vi "Apply Theme To Buttons.vi"(7 "Override Root With (Empty)":string, 8 "Error In":errorcluster, 9 "Window Element":T1, 10 "Buttons Ref":refnum<vi>[](array[refnum]), 11 "ini Theme in":refnum<class "ini Theme.lvclass">) -> (0 "Error Out":errorcluster, 3 "ini Theme out":refnum<class "ini Theme.lvclass">)   [LabVIEW 2021, in "Appearance Actor.lvlib" / "ini Theme.lvclass"]
doc: "Apply theme to <B>Buttons</B> (Bool Reference Array). <B>Window Element</B> enum tells where it is on the window. <B>Override Root With</B> allows to override styling used for main window components."
uses:
  ini Theme.lvclass
  Generic Theme/API/Typedefs/Window Element--enum.ctl
  Generic Theme/API/Typedefs/Theme Control Property--enum.ctl
  ini Theme.lvclass/ini Theme.ctl
  f5176d82-9832-41ee-acb3-f85e09ee67a5.vi
  f5176d82-9832-41ee-acb3-f85e09ee67a5.vi/e124eda1-1651-4d76-919f-d33a8200b27b.vi
  f5176d82-9832-41ee-acb3-f85e09ee67a5.vi/2055fcb7-c480-499a-9c31-028cc01b484e.vi
  Generic Theme/API/Utilities/Theme Entry Enum To String.vi
  Generic Theme/API/Utilities/U32 Color To Hexa String.vi
  <vilib>/Utility/config.llb/Read Key.vi
  <vilib>/Utility/config.llb/Read Key (String).vi
  <vilib>/Utility/config.llb/NI_LVConfig.lvlib
  Generic Theme/Generic Theme.lvclass
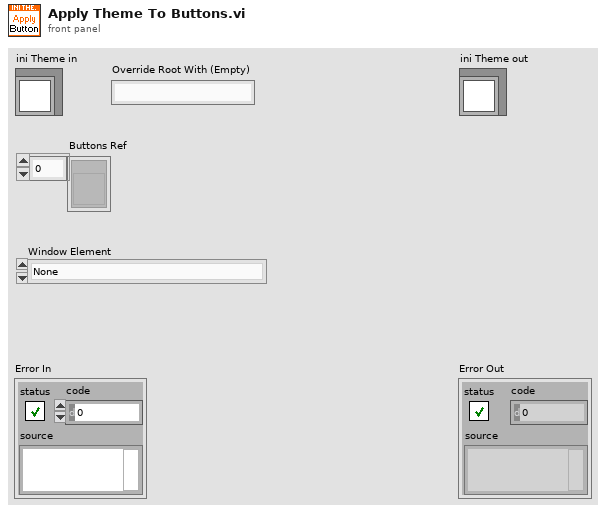
[diagram p1: front panel]
types:
  T1 = typedef "Appearance Actor.lvlib/Generic Theme.lvclass/Window Element--enum.ctl" = enum16{"None", "TB", "SM", "BP", "SB"}
  T2 = typedef "Appearance Actor.lvlib/Generic Theme.lvclass/Theme Control Property--enum.ctl" = enum16{"None", "Button.FalseFillColor", "Button.FalseOutlineColor", "Button.FalseToTrueFillColor", "Button.FalseToTrueOutlineColor", "Button.HoverFalseFillColor", "Button.HoverFalseOutlineColor", "Button.HoverTrueFillColor", "Button.HoverTrueOutlineColor", "Button.TrueFillColor", "Button.TrueOutlineColor", "Button.TrueToFalseFillColor", "Button.TrueToFalseOutlineColor", "CloseButton.FalseFillColor", "CloseButton.FalseOutlineColor", "CloseButton.FalseToTrueFillColor", "CloseButton.FalseToTrueOutlineColor", "CloseButton.HoverFalseFillColor", "CloseButton.HoverFalseOutlineColor", "CloseButton.HoverTrueFillColor", "CloseButton.HoverTrueOutlineColor", "CloseButton.TrueFillColor", "CloseButton.TrueOutlineColor", "CloseButton.TrueToFalseFillColor", "CloseButton.TrueToFalseOutlineColor", "Pane.Color", "Splitter.FillColor", "Splitter.OutlineColor", "Splitter.Size", "Title.Font.Color", "Title.Font.Family", "Title.Font.Size", "Title.Font.Style"}
  T3 = typedef "NI_LVConfig.lvlib/Config Data RefNum.ctl" = refnum<k1>
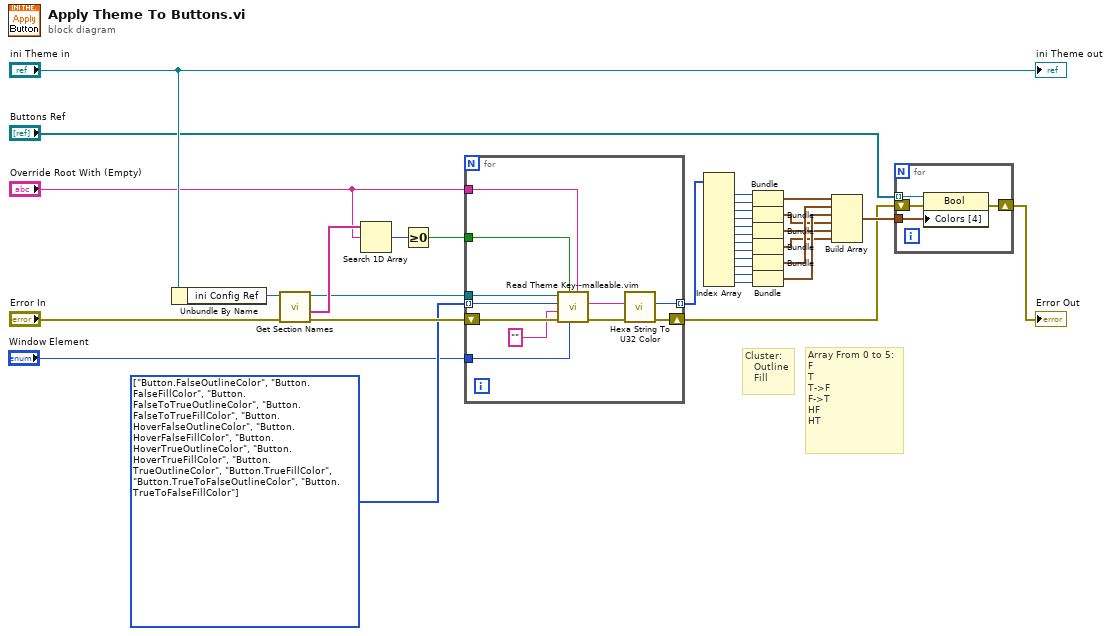
[diagram p0: block diagram]
diagram:
  w25 = T2[] [enum."Button.FalseOutlineColor", enum."Button.FalseFillColor", enum."Button.FalseToTrueOutlineColor", enum."Button.FalseToTrueFillColor", enum."Button.HoverFalseOutlineColor", enum."Button.HoverFalseFillColor", enum."Button.HoverTrueOutlineColor", enum."Button.HoverTrueFillColor", enum."Button.TrueOutlineColor", enum."Button.TrueFillColor", enum."Button.TrueToFalseOutlineColor", enum."Button.TrueToFalseFillColor"] items=["None", "Button.FalseFillColor", "Button.FalseOutlineColor", "Button.FalseToTrueFillColor", "Button.FalseToTrueOutlineColor", "Button.HoverFalseFillColor", "Button.HoverFalseOutlineColor", "Button.HoverTrueFillColor", "Button.HoverTrueOutlineColor", "Button.TrueFillColor", "Button.TrueOutlineColor", "Button.TrueToFalseFillColor", "Button.TrueToFalseOutlineColor", "CloseButton.FalseFillColor", "CloseButton.FalseOutlineColor", "CloseButton.FalseToTrueFillColor", "CloseButton.FalseToTrueOutlineColor", "CloseButton.HoverFalseFillColor", "CloseButton.HoverFalseOutlineColor", "CloseButton.HoverTrueFillColor", "CloseButton.HoverTrueOutlineColor", "CloseButton.TrueFillColor", "CloseButton.TrueOutlineColor", "CloseButton.TrueToFalseFillColor", "CloseButton.TrueToFalseOutlineColor", "Pane.Color", "Splitter.FillColor", "Splitter.OutlineColor", "Splitter.Size", "Title.Font.Color", "Title.Font.Family", "Title.Font.Size", "Title.Font.Style"] ("Array")
  # "Cluster:\n   Outline\n   Fill"
  # "Array From 0 to 5:\nF\nT\nT->F\nF->T\nHF\nHT"
  n1 = Unbundle By Name("ini Theme in") -> ("ini Config Ref"=w34:T3)
  n2 = call <vilib>:"Get Section Names.vi"("error in (no error)"="Error In", "refnum"=w34) -> ("error out"=w31:errorcluster, "section names"=w33:string[], "refnum out"=w26:T3)  [unwired: 7 in]
  n3 = Search 1D Array(1D array=w33, element="Override Root With (Empty)") -> (index of element=w32:i32)  [unwired: 1 in]
  n4 = Greater Or Equal To 0?(x=w32) -> (x >= 0?=w27:bool)
  n5 = for {
    shift-right: [w36] -> w3
    shift-left: w31 -> [w44]
    tunnel: "Override Root With (Empty)" -> [w43]
    tunnel: w27 -> [w42]
    tunnel: w26 -> [w41]
    tunnel: w25 -> [w40] mode=indexing
    tunnel: "Window Element" -> [w39]
    tunnel: [w35] -> w23 mode=indexing
    n6 = call "Read Theme Key--malleable.vim"("Section for Override (Empty)"=w43, "Window Element"=w39, "Can Be Overriden (F)"=w42, "Error In"=w44, "Data Type"="", "Theme Control Property"=w40, "ini Ref In"=w41) -> ("Error Out"=w36:errorcluster, "Value"=w37:string)  [unwired: 2 in, 1 out]
    n7 = call "Hexa String To U32 Color.vi"("8 Char Hexa String"=w37) -> ("U32 Color"=w35:u32)  [unwired: 10 in]
  }
  n8 = Index Array(array=w23) -> (element #1=w21:u32, element #2=w22:u32, element #3=w20:u32, element #4=w19:u32, element #5=w18:u32, element #6=w17:u32, element #7=w16:u32, element #8=w15:u32, element #9=w14:u32, element #10=w13:u32, element #11=w12:u32, element #12=w11:u32)  [unwired: 12 in]
  n9 = Bundle("U32 Color"=w21, "U32 Color"=w22) -> (w10:cluster{"U32 Color":u32, "U32 Color":u32})  [unwired: 1 in]
  n10 = Bundle("U32 Color"=w20, "U32 Color"=w19) -> (w7:cluster{"U32 Color":u32, "U32 Color":u32})  [unwired: 1 in]
  n11 = Bundle("U32 Color"=w18, "U32 Color"=w17) -> (w6:cluster{"U32 Color":u32, "U32 Color":u32})  [unwired: 1 in]
  n12 = Bundle("U32 Color"=w16, "U32 Color"=w15) -> (w5:cluster{"U32 Color":u32, "U32 Color":u32})  [unwired: 1 in]
  n13 = Bundle("U32 Color"=w14, "U32 Color"=w13) -> (w9:cluster{"U32 Color":u32, "U32 Color":u32})  [unwired: 1 in]
  n14 = Bundle("U32 Color"=w12, "U32 Color"=w11) -> (w8:cluster{"U32 Color":u32, "U32 Color":u32})  [unwired: 1 in]
  n15 = Build Array(w10, w9, w8, w7, w6, w5) -> (w4:cluster{"U32 Color":u32, "U32 Color":u32}[])
  n16 = for {
    tunnel: w4 -> [w48]
    tunnel: "Buttons Ref" -> [w45] mode=indexing
    shift-right: [w46] -> w2
    shift-left: w3 -> [w47]
    n17 = property class="Bool"(reference=w45, error in=w47, "Colors [4]"=w48) -> (error out=w46:errorcluster)  [unwired: 1 out]
  }
  "Error Out" <- w2
  "ini Theme out" <- "ini Theme in"
